vi "Stopwatch.vi"(7 "ms":u32, 8 "Load":bool, 9 "Reset":bool, 10 "Start":bool) -> (2 "t ms":u32, 3 "End":bool)   [LabVIEW 2019, in "Timers.lvlib"]
uses:
  Timers.lvlib
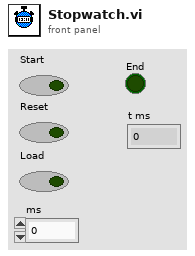
[diagram p1: front panel]
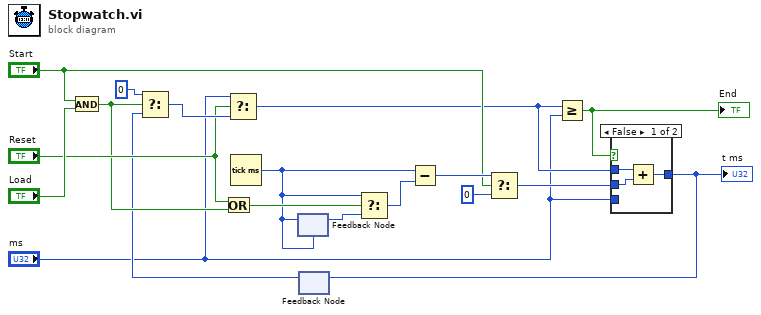
[diagram p0: block diagram]
diagram:
  n1 = And(x="Start", y="Load") -> (x .and. y?=w13:bool)
  n2 = Or(x="Reset", y=w13) -> (x .or. y?=w17:bool)
  n3 = Tick Count (ms)() -> (millisecond timer value=w4:u32)
  n4 = feedback #1(w4) -> (w18:u32)
  n5 = feedback-in #1(w4) -> ()
  n6 = feedback #2() -> (w11:u32)  [unwired: 1 in]
  n7 = Select(t=u32 0, s=w13, f=w11) -> (s? t:f=w15:u32)
  n8 = Select(t="ms", s="Reset", f=w15) -> (s? t:f=w2:u32)
  n9 = Select(t=w4, s=w17, f=w18) -> (s? t:f=w5:u32)
  n10 = Subtract(x=w4, y=w5) -> (x-y=w9:u32)
  n11 = Select(t=w9, s="Start", f=u32 0) -> (s? t:f=w6:u32)
  n12 = Greater Or Equal?(x=w2, y="ms") -> (x >= y?=w12:bool)
  "End" <- w12
  n13 = case shown="False" w12 {
    tunnel: w6 -> [w20 _]
    tunnel: [w21 w22] -> w10
    tunnel: w2 -> [w19 _]
    tunnel: "ms" -> [_ w22]
    frame False {
      n14 = Add(x=w19, y=w20) -> (x+y=w21:u32)
    }
    frame True {
    }
  }
  "t ms" <- w10
  n15 = feedback-in #2(w10) -> ()
